vi "Module Type.vi"(11 "Telemetry Client in":refnum<class "Telemetry Client.lvclass">) -> (2 "Module Type":string)   [LabVIEW 2020, in "VolatusTelemetry.lvlib" / "Telemetry Client.lvclass"]
uses:
  Telemetry Client.lvclass
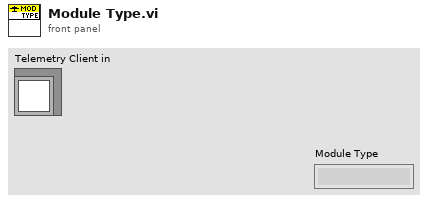
[diagram p1: front panel]
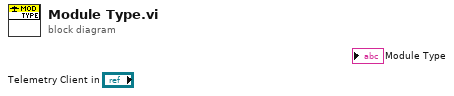
[diagram p0: block diagram]
diagram:
